vi "Get Plugin gRPC ID.vi"(8 "error in (no error)":errorcluster, 9 "Plugin Name":string, 10 "Index":i32, 11 "CIF_UI in":refnum<class "CIF_UI.lvclass">) -> (0 "error out":errorcluster, 1 "Not Found":bool, 2 "gRPC ID":T1, 3 "CIF_UI out":refnum<class "CIF_UI.lvclass">)   [LabVIEW 2021, in "CIF_UI.lvclass"]
uses:
  CIF_UI.lvclass
  <vilib>/gRPC/LabVIEW gRPC Library/Shared/grpcId.ctl
  CIF_UI.lvclass/CIF_UI.ctl
  Accessors/Read Plugin Connection Map.vi
  <vilib>/gRPC/LabVIEW gRPC Library/grpc-lvsupport-release.lvlib
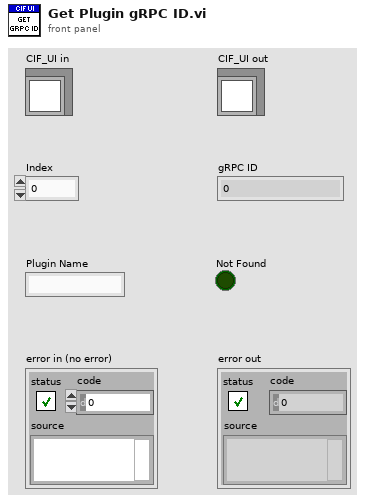
[diagram p1: front panel]
types:
  T1 = typedef "grpc-lvsupport-release.lvlib/grpcId.ctl" = u64
  T2 = typedef "CIF_UI.lvclass/Plugin Connection Map.ctl" = map{string, T3}
  T3 = typedef "CIF_UI.lvclass/Plugin Connections.ctl" = cluster{"gRPC ID":T1, "Plugin Info":T4}
  T4 = typedef "CIF_UI.lvclass/PluginInfo.ctl" = cluster{"Name":string, "Type":string, "grpc_port":i32, "Version":T5, "Node Status":T6}
  T5 = typedef "CIF_UI.lvclass/Version.ctl" = cluster{"Major":i32, "Minor":i32, "Fix":i32}
  T6 = typedef "CIFCoreCommon.lvlib/gRPC Reported Plugin Status.ctl" = cluster{"State":T7, "Timing Statistics (us)":T8, "FIFO Statistics (us)":T10, "error":T11, "Monitor Doubles":T12, "Monitor U64":T13, "Monitor I64":T14}
  T7 = typedef "CIFCoreCommon.lvlib/Plugin State.ctl" = enum32{"Null", "Creating", "Listening", "Running", "CleaningUp", "Destroying"}
  T8 = typedef "CIFCoreCommon.lvlib/Timing Statistics.ctl" = cluster{"Period":T9, "Wake Error":T9, "Execute":T9, "Housekeep":T9, "Idle":T9, "Cleanup":T9, "Custom 1 (custom units)":T9, "Custom 2 (custom units)":T9}
  T9 = typedef "CIFCoreCommon.lvlib/Timing Stats Base.ctl" = cluster{"Max":i64, "Avg":dbl, "Min":i64}
  T10 = typedef "CIFCoreCommon.lvlib/FIFO Statistics.ctl" = cluster{"From T0":T9, "From Previous Plugin":T9, "Output Error":T9}
  T11 = typedef "CIFCoreCommon.lvlib/Simple Error.ctl" = cluster{"status":bool, "code":i32}
  T12 = typedef "CIFCoreCommon.lvlib/Monitor Doubles.ctl" = cluster{"1":dbl, "2":dbl, "3":dbl, "4":dbl}
  T13 = typedef "CIFCoreCommon.lvlib/Monitor U64.ctl" = cluster{"1":u64, "2":u64, "3":u64, "4":u64}
  T14 = typedef "CIFCoreCommon.lvlib/Monitor I64.ctl" = cluster{"1":i64, "2":i64, "3":i64, "4":i64}
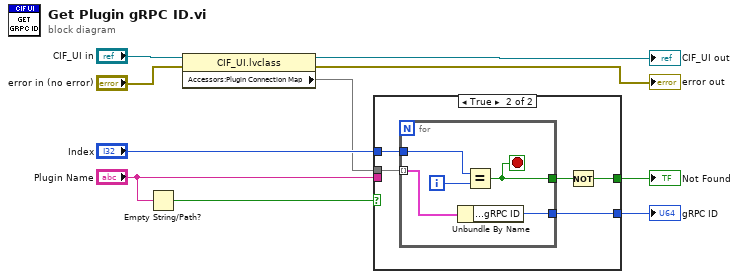
[diagram p0: block diagram]
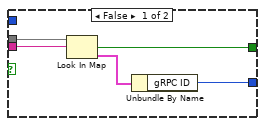
[diagram p2: hidden frame]
diagram:
  n1 = Empty String/Path?(string/path="Plugin Name") -> (empty?=w10:bool)
  n2 = property class="CIF_UI.lvclass"(reference="CIF_UI in", error in="error in (no error)") -> (reference out=→"CIF_UI out":refnum<class "CIF_UI.lvclass">, error out=→"error out":errorcluster, "Accessors:Plugin Connection Map"=w5:T2)
  n3 = case shown="True" w10 {
    tunnel: w5 -> [w15 w20]
    tunnel: "Plugin Name" -> [w14 _]
    tunnel: [w13 w16] -> w8
    tunnel: [w11 w18] -> w7
    tunnel: "Index" -> [_ w19]
    frame False {
      n4 = Look In Map(map=w15, key=w14) -> (key not found?=w13:bool, value=w12:T3)  [unwired: 1 in]
      n5 = Unbundle By Name(w12) -> ("gRPC ID"=w11:T1)
    }
    frame True {
      n6 = for {
        tunnel: w20 -> [w25] mode=indexing
        tunnel: w19 -> [w24]
        tunnel: [w22] -> w18
        tunnel: [w21] -> w17
        i -> [w23]
        stop <- w21 stop-if-true
        n7 = Unbundle By Name(w25) -> ("Plugin Connections.gRPC ID"=w22:T1)
        n8 = Equal?(x=w24, y=w23) -> (x = y?=w21:bool)
      }
      n9 = Not(x=w17) -> (.not. x?=w16:bool)
    }
  }
  "Not Found" <- w8
  "gRPC ID" <- w7
